vi "FGVSafeTip.vi"(7 "Enum":T2, 8 "error in":errorcluster, 9 "SafeTipOn?":bool, 10 "SafeTipParametersIn":T1 {"SafeTipSignal" items=["AI0", "AI1", "AI2", "AI3", "AI4", "AI5", "AI6", "AI7"]}) -> (0 "error out":errorcluster, 1 "SafeTipOn?":bool, 2 "SafeTipParametersOut":T1 {"SafeTipSignal" items=["AI0", "AI1", "AI2", "AI3", "AI4", "AI5", "AI6", "AI7"]})   [LabVIEW 2016]
uses:
  controls/Enum.ctl
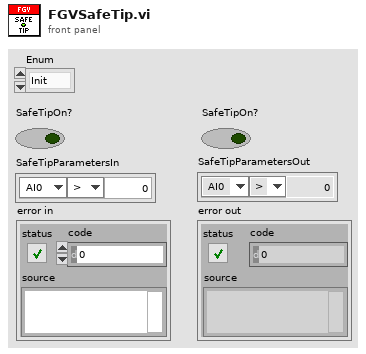
[diagram p1: front panel]
types:
  T1 = cluster{"SafeTipValue":dbl, ">/<":enum16{">", "<"}, "SafeTipSignal":u16}
  T2 = typedef "Enum.ctl" = enum16{"Init", "Read", "Write"}
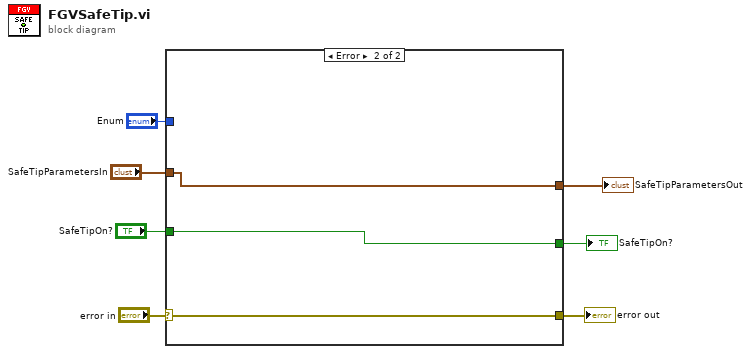
[diagram p0: block diagram]
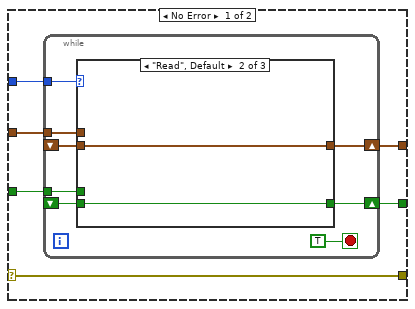
[diagram p2: hidden frame]
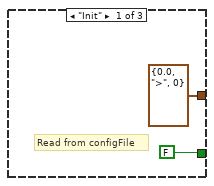
[diagram p3: hidden frame]
diagram:
  n1 = case shown="Error" "error in" {
    selector: "error in" -> [w12 w30]
    tunnel: "Enum" -> [w13 _]
    tunnel: [w12 w30] -> w6
    tunnel: "SafeTipOn?" -> [w11 w29]
    tunnel: [w10 w29] -> w3
    tunnel: "SafeTipParametersIn" -> [w9 w28]
    tunnel: [w8 w28] -> w1
    frame No Error {
      n2 = while {
        tunnel: w13 -> [w20]
        tunnel: w11 -> [w19]
        shift-right: [w18] -> w10
        shift-left: _ -> [w17]
        tunnel: w9 -> [w16]
        shift-right: [w15] -> w8
        shift-left: _ -> [w14]
        stop <- TRUE stop-if-true
        n3 = case shown="\"Read\", Default" w20 {
          tunnel: w19 -> [_ _ w27]
          tunnel: [FALSE w25 w27] -> w18
          tunnel: w17 -> [_ w25 _]
          tunnel: w16 -> [_ _ w26]
          tunnel: [T1 {"SafeTipValue"=0.0, ">/<"=enum.">", "SafeTipSignal"=0} ("SafeTipParametersIn") w24 w26] -> w15
          tunnel: w14 -> [_ w24 _]
          frame "Init" {
            # "Read from configFile"
          }
          frame "Read", Default {
          }
          frame "Write" {
          }
        }
      }
    }
    frame Error {
    }
  }
  "error out" <- w6
  "SafeTipOn?" <- w3
  "SafeTipParametersOut" <- w1
